vi "Thermometer.vi"(1 "Temp Scale":bool) -> (0 "Temperature":dbl(slide) scale=0.0..100.0)   [LabVIEW 2020]
doc: "This VI measures temperature using the temperature sensor on the DAQ Signal Accessory."
panel:
  # "deg C"
  # "deg F"
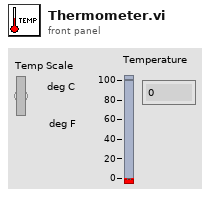
[diagram p1: front panel]
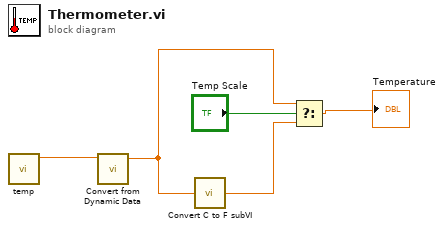
[diagram p0: block diagram]
diagram:
  n1 = call "temp.vi"() -> ("voltage"=w1:dbl)  [unwired: 6 in, 1 out]
  n2 = call "Convert from Dynamic Data"("Dynamic Data Type"=w1) -> ("Scalar"=w2:dbl)  [unwired: 3 in]
  n3 = call "Convert C to F subVI.vi"("deg C"=w2) -> ("deg F"=w3:dbl)
  n4 = Select(t=w2, s="Temp Scale", f=w3) -> (s? t:f=→"Temperature":dbl)
